vi "Wait For Response.vi"(8 "error in (no error)":errorcluster, 9 "timeout in ms (0)":i32, 11 "Interface in":refnum<class "Interface.lvclass">) -> (0 "error out":errorcluster, 1 "timed out?":bool, 2 "response data":u8[](array[numeric]), 3 "Interface out":refnum<class "Interface.lvclass">, 4 "# elements":u32)   [LabVIEW 2021, in "DSF Core.lvlib" / "Interface.lvclass"]
uses:
  Interface.lvclass
  Interface.lvclass/Interface.ctl
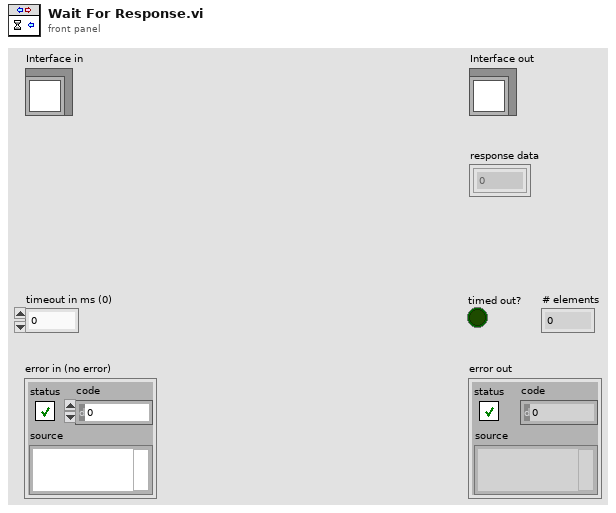
[diagram p1: front panel]
types:
  T1 = typedef "DSF Core.lvlib/Framework.lvclass/DSF FIFO Options.ctl" = cluster{"Infinite Timeouts":bool}
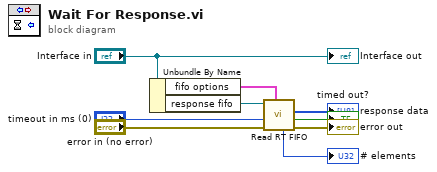
[diagram p0: block diagram]
diagram:
  n1 = Unbundle By Name("Interface in") -> ("fifo options"=w2:T1, "response fifo"=w3:refnum<k33>)
  n2 = call "Read RT FIFO.vi"("fifo options"=w2, "error in (no error)"="error in (no error)", "timeout in ms (0)"="timeout in ms (0)", "rt fifo in"=w3) -> ("error out"=→"error out":errorcluster, "empty?"=→"timed out?":bool, "element"=→"response data":u8[], "# elements"=→"# elements":u32)  [unwired: 3 in, 1 out]
  "Interface out" <- "Interface in"
